vi "SGUI Assign Multiple Strings With Tags.vi"(6 "error in":errorcluster, 8 "string refs":refnum<vi>[](array[refnum]), 9 "string (empty)":string, 10 "keep last font face setup (False)":bool) -> (7 "error out":errorcluster, 11 "string refs out (copy)":refnum<vi>[](array[refnum]))   [LabVIEW 2013, in "varilib.lvlib"]
doc: "This is multiline version of tag formatted text writter. When more than one reference is entered the 'string' is parsed to lines. Each line is assigned to one of the referenced string objects. If there are more lines of text than references the rest of the 'string' is assigned to the last referenced string object.\n\nFor format details see the single control version.\n\nKeep in mind the format tags applies always only for one line (one referenced string object). So when multiple lines are to have the same format the tags must be repeated for each line!\n\nThis VI ignores input error (will execute anyway) however will generate error if writting any of the references fails (invalid reference)."
uses:
  varilib.lvlib
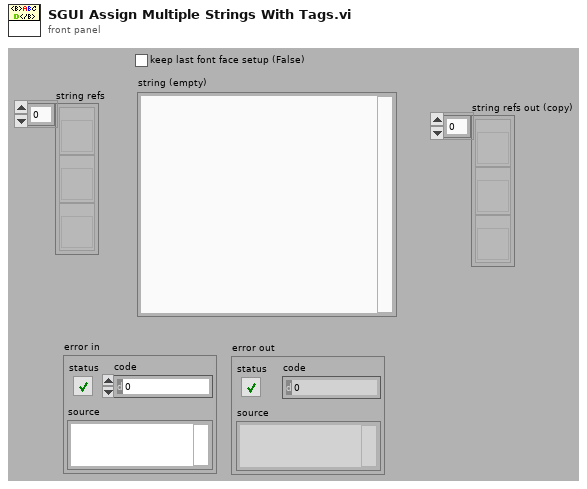
[diagram p1: front panel]
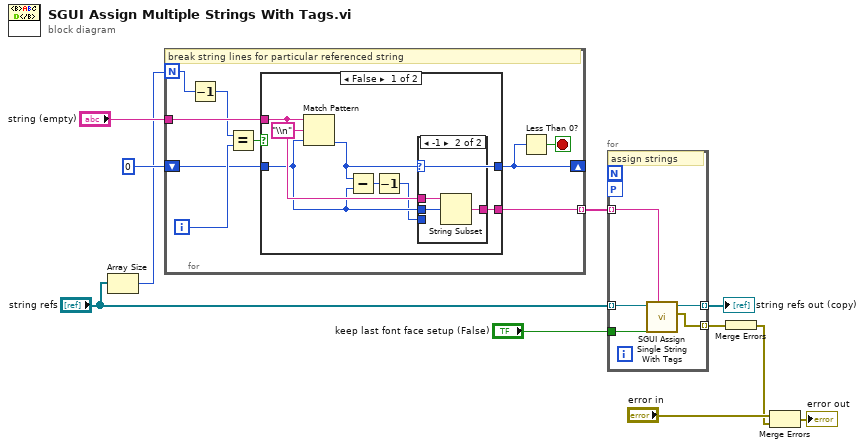
[diagram p0: block diagram]
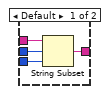
[diagram p2: hidden frame]
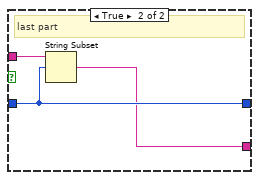
[diagram p3: hidden frame]
diagram:
  n1 = Array Size(array="string refs") -> (size(s)=w6:i32)
  n2 = for {
    N: w6 -> [w17]
    tunnel: "string (empty)" -> [w20]
    shift-right: [w12] -> _
    shift-left: 0 -> [w15]
    tunnel: [w14] -> w9 mode=indexing
    i -> [w18]
    stop <- w13 stop-if-true
    # "break string lines for particular referenced string"
    n3 = Decrement(x=w17) -> (x-1=w16:i32)
    n4 = Equal?(x=w16, y=w18) -> (x = y?=w19:bool)
    n5 = case shown="False" w19 {
      tunnel: w20 -> [w25 w37]
      tunnel: w15 -> [w24 w36]
      tunnel: [w26 w35] -> w14
      tunnel: [w21 w36] -> w12
      frame False {
        n6 = Match Pattern(string=w25, regular expression="\\n", offset (0)=w24) -> (offset past match=w21:i32)  [unwired: 3 out]
        n7 = Subtract(x=w21, y=w24) -> (x-y=w27:i32)
        n8 = Decrement(x=w27) -> (x-1=w22:i32)
        n9 = case shown="-1" w21 {
          tunnel: [w31 w34] -> w26
          tunnel: w25 -> [w30 w33]
          tunnel: w24 -> [w29 w32]
          tunnel: w22 -> [w28 _]
          frame Default {
            n10 = String Subset(string=w30, offset (0)=w29, length (rest)=w28) -> (substring=w31:string)
          }
          frame -1 {
            n11 = String Subset(string=w33, offset (0)=w32) -> (substring=w34:string)  [unwired: 1 in]
          }
        }
      }
      frame True {
        # "last part"
        n12 = String Subset(string=w37, offset (0)=w36) -> (substring=w35:string)  [unwired: 1 in]
      }
    }
    n13 = Less Than 0?(x=w12) -> (x < 0?=w13:bool)
  }
  n14 = for {
    tunnel: "string refs" -> [w42] mode=indexing
    tunnel: [w41] -> w8 mode=indexing
    tunnel: w9 -> [w40] mode=indexing
    tunnel: "keep last font face setup (False)" -> [w39]
    workers-P: _ -> [_]
    tunnel: [w38] -> w4 mode=indexing
    # "assign strings"
    n15 = call "SGUI Assign Single String With Tags.vi"("string ref"=w42, "string (empty)"=w40, "keep last font face setup (False)"=w39) -> ("error out"=w38:errorcluster, "string ref out (copy)"=w41:refnum<vi>)  [unwired: 7 in]
  }
  "string refs out (copy)" <- w8
  n16 = Merge Errors(w4) -> (w2:errorcluster)
  n17 = Merge Errors("error in", w2) -> (→"error out":errorcluster)
